vi "test Import To Empty Module Same Slot.vi"(8 "error in (no error)":errorcluster, 11 "TestCase in":refnum<class "SLSC Switch Import Export Unit Tests.lvclass">) -> (0 "error out":errorcluster, 3 "TestCase out":refnum<class "SLSC Switch Import Export Unit Tests.lvclass">)   [LabVIEW 2017, in "SLSC Switch Import Export Unit Tests.lvclass"]
uses:
  SLSC Switch Import Export Unit Tests.lvclass
  Shared/Endpoint Configuration Cluster.ctl
  Shared/Endpoint Configuration Enum.ctl
  SLSC Switch Import Export Unit Tests.lvclass/SLSC Switch Import Export Unit Tests.ctl
  <vilib>/addons/_JKI Toolkits/VI Tester/TestCase.llb/TestCase.lvclass
  <vilib>/NI/NI VeriStand Custom Device Import and Export Tool/ImportExport.lvlib
  Scripting/SLSC Switch Scripting.lvlib
  Shared/VeriStand System Definition Test Utilities/VeriStand System Definition Test Utilities.lvlib
  Shared/SLSC Switch Shared.lvlib
  C:/Program Files (x86)/National Instruments/LabVIEW 2017/vi.lib/addons/_JKI Toolkits/VI Tester/TestCase.llb/TestCase.lvclass
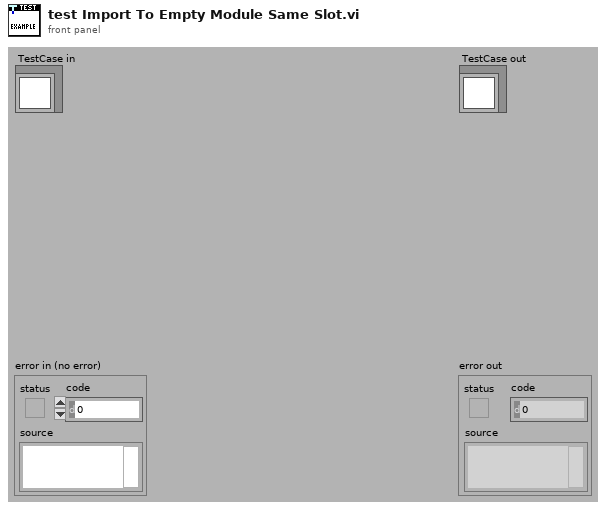
[diagram p1: front panel]
types:
  T1 = cluster{"Ignore Properties":string[], "Ignore Top Level Name":bool}
  T2 = typedef "SLSC Switch Shared.lvlib/Endpoint Configuration Cluster.ctl" = cluster{"Endpoint":string, "Configuration":T3}
  T3 = typedef "SLSC Switch Shared.lvlib/Endpoint Configuration Enum.ctl" = enum16{"Load", "Source", "Configuration"}
  T4 = typedef "Custom Device API.lvlib/Custom Device Item Ref.ctl" = u64
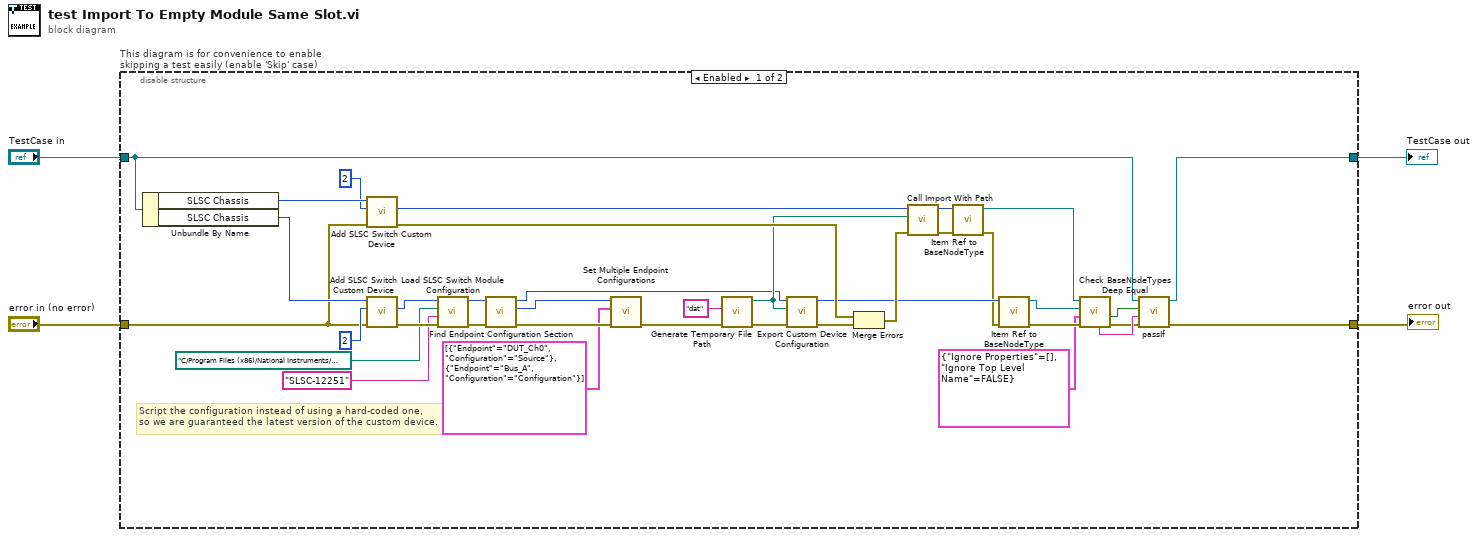
[diagram p0: block diagram]
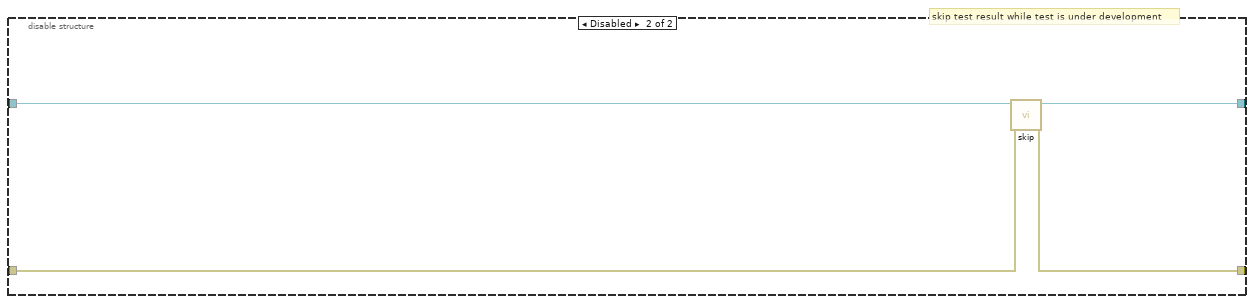
[diagram p2: hidden frame]
diagram:
  n1 = disable-structure "This diagram is for convenience to enable skipping a test easily (enable 'Skip' case)" shown="Enabled" {
    disable-tunnel: "TestCase in" -> [w27 w45]
    disable-tunnel: [w6 w43] -> w1
    disable-tunnel: [w5 w44] -> w3
    disable-tunnel: "error in (no error)" -> [w21 w42]
    frame Enabled {
      # "Script the configuration instead of using a hard-coded one,\nso we are guaranteed the latest version of the custom device."
      n2 = Unbundle By Name(w27) -> ("SLSC Chassis"=w22:u64, "SLSC Chassis"=w41:u64)
      n3 = call "Add SLSC Switch Custom Device.vi"("error in"=w21, "slot number"=u32 2, "slsc chassis in"=w22) -> ("error out"=w36:errorcluster, "slsc switch custom device"=w7:T4)  [unwired: 6 in, 1 out]
      n4 = call "Add SLSC Switch Custom Device.vi"("error in"=w21, "slot number"=u32 2, "slsc chassis in"=w41) -> ("error out"=w20:errorcluster, "slsc switch custom device"=w18:T4)  [unwired: 6 in, 1 out]
      n5 = call "Load SLSC Switch Module Configuration.vi"("error in"=w20, "product name"="SLSC-12251", "switches json file"=path "C:/Program Files (x86)/National Instruments/Shared/NI-SLSC Switch/Modules/SLSC-12251-switches.json", "slsc switch custom device in"=w18) -> ("error out"=w19:errorcluster, "slsc switch custom device out"=w14:T4)  [unwired: 6 in]
      n6 = call "Find Endpoint Configuration Section.vi"("error in"=w19, "slsc switch custom device in"=w14) -> ("error out"=w15:errorcluster, "endpoint configuration"=w12:T4, "slsc switch custom device out"=w11:T4)  [unwired: 7 in]
      n7 = call "Set Multiple Endpoint Configurations.vi"("error in"=w15, "endpoint configurations"=T2[] [{"Endpoint"="DUT_Ch0", "Configuration"=enum."Source"}, {"Endpoint"="Bus_A", "Configuration"=enum."Configuration"}], "endpoint configuration in"=w12) -> ("error out"=w13:errorcluster)  [unwired: 7 in, 1 out]
      n8 = call <vilib>:"Generate Temporary File Path.vi"("error in (no error)"=w13, "Temporary File Extension (tmp)"="dat") -> ("error out"=w38:errorcluster, "Unique Temporary File Path"=w34:path)  [unwired: 8 in]
      n9 = call <vilib>:"Export Custom Device Configuration.vi"("error in (no error)"=w38, "Path"=w34, "ID"=w11) -> ("error out"=w37:errorcluster, "ID out"=w32:u64)  [unwired: 7 in]
      n10 = Merge Errors(w36, w37) -> (w35:errorcluster)
      n11 = call "Call Import With Path.vi"("error in (no error)"=w35, "Path"=w34, "Node Ptr"=w7) -> ("error out"=w31:errorcluster, "Node Ptr out"=w33:u64)  [unwired: 7 in]
      n12 = call "Item Ref to BaseNodeType.vi"("error in (no error)"=w31, "Item Ref"=w33) -> ("error out"=w30:errorcluster, "BaseNodeType"=w24:refnum<k24>)  [unwired: 8 in]
      n13 = call "Item Ref to BaseNodeType.vi"("error in (no error)"=w30, "Item Ref"=w32) -> ("error out"=w29:errorcluster, "BaseNodeType"=w28:refnum<k24>)  [unwired: 8 in]
      n14 = call "Check BaseNodeTypes Deep Equal.vi"("error in (no error)"=w29, "Settings"=T1 {"Ignore Properties"=[], "Ignore Top Level Name"=FALSE}, "BaseNodeType 2"=w28, "BaseNodeType 1"=w24) -> ("error out"=w23:errorcluster, "Equal?"=w26:bool, "Inequality context"=w25:string)  [unwired: 3 in, 2 out]
      n15 = call-dynamic "passIf.vi"("error in (no error)"=w23, "message (\"\")"=w25, "pass"=w26, "TestCase in"=w27) -> ("error out"=w5:errorcluster, "TestCase out"=w6:refnum<class "SLSC Switch Import Export Unit Tests.lvclass">)  [unwired: 6 in]
    }
    frame Disabled {
      # "skip test result while test is under development"
      n16 = call <vilib>:"skip.vi"("error in (no error)"=w42, "TestCase in"=w45) -> ("error out"=w44:errorcluster, "TestCase out"=w43:refnum<class "SLSC Switch Import Export Unit Tests.lvclass">)  [unwired: 8 in]
    }
  }
  "error out" <- w3
  "TestCase out" <- w1
